vi "AnalogIntegrator_NI5751.vi"() -> ()   [LabVIEW 2012]
uses:
  <vilib>/Platform/TimedLoop/XDataNode/timing_clust.ctl
  <vilib>/Platform/TimedLoop/XDataNode/nitl_modes.ctl
  <vilib>/Platform/TimedLoop/XDataNode/wakeup.ctl
  <vilib>/rvi/eio/common/nirviEmuTemplateMethod_errors.vi
  <vilib>/rvi/FIFO/Fifo_Resource/nirvififoEmulationSetSize.vi
  <vilib>/rvi/DataTransferAndStorage/Container/Common/niFpgaContainerGetUniqueNameForEmu.vi
  <vilib>/rvi/Emulation/niFpgaSctlEmulationRegisterWithScheduler.vi
  <vilib>/rvi/errors/niFpgaSetErrorForExecOnDevCompSimple.vi
  <vilib>/rvi/eio/common/nirviEmuReportErrorAndStop.vi
  <vilib>/rvi/Emulation/niFpgaSctlEmulationFifoFullMgr.vi
  <vilib>/rvi/Emulation/niFpgaSctlEmulationResourceMgr.vi
  <vilib>/rvi/Emulation/niFpgaSctlEmulationScheduler.vi
  <vilib>/rvi/interface/RandomDataEmulation/nirviRandomDataFPGAFIFO.vi
  <vilib>/rvi/interface/RandomDataEmulation/niFpgaRandomDataHandleErrors.vi
  <vilib>/rvi/Emulation/niFpgaSctlEmulationGlobalWrite.vi
  <vilib>/Platform/TimedLoop/XDataNode/XDataNode.xnode
  <vilib>/eio/EIONode/EIONode.xnode
  <vilib>/rvi/DataTransferAndStorage/Container/XNode/niFpgaContainer.xnode
  <vilib>/rvi/FIFO/Fifo_Resource/nirvififoEmulationClear.vi
  <vilib>/rvi/FIFO/Fifo_Resource/nirvififoEmulationWrite.vi
  <vilib>/rvi/FIFO/Fifo_Resource/nirvififoEmulationRead.vi
  <vilib>/rvi/interface/RandomDataEmulation/nirviRandomDataFpgaReadWriteTemplate.vi
  <vilib>/Platform/TimedLoop/XDataNode/XDNodeRunTimeDep.lvlib
panel:
  in  "Baselinex8 Ch2":u16
  in  "Baselinex8 Ch1":u16
  in  "Clear Interloop FIFO":bool
  out "InterloopFIFO Timeout":bool
  out "ToHostCh2FIFO Overflow":bool
  out "ToHostCh1FIFO Overflow":bool
  out "Pixel counter":u32
  in  "Wait for trigger":bool
  in  "Acquire":bool
  in  "Acquire continuously":bool=TRUE
  in  "Requested pixels":u32=100000
  out "InterloopFIFO Overflow":bool
  out "Acquiring":bool
  out "IO Module\\AI Over Range":bool
  in  "Samples per pixel":u32=10000 caption="Samples per pixel Acq"
  in  "Samples per line":u32=10000 caption="Samples per pixel Acq"
  out "Configured?":bool
  # "5771 IO module configuration"
  # "Analog integrator"
  # "Acquisition control"
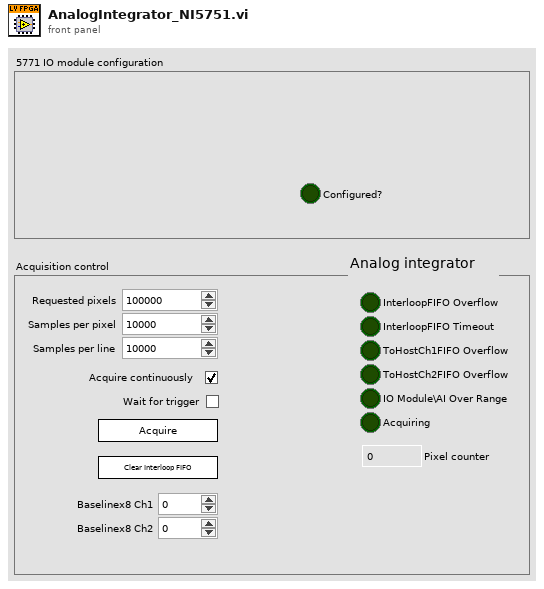
[diagram p1: front panel]
types:
  T1 = typedef "XDNodeRunTimeDep.lvlib/timing_clust.ctl" = cluster{"Expected End [f-1]":u64, "Actual End [f-1]":u64, "Finished Late? [f-1]":bool, "Expected End [i-1]":u64, "Actual End [i-1]":u64, "Finished Late? [i-1]":bool, "Expected Start [i]":u64, "Actual Start [i]":u64, "Expected Start [f]":u64, "Actual Start [f]":u64, "Source Name":string, "Structure Name":string, "Period":i64, "Deadline":i64, "Offset":i64, "Start":i64, "Priority":i32, "Timeout":i32, "Mode":T2, "Wakeup Reason":T3, "Error":errorcluster, "Source Type":string, "Secondary Source Type":string, "Global End Time":u64, "Global Start Time":u64, "Frame Duration":u64, "Iteration Duration":u64, "Assigned CPU":i32, "I/O Scan Engine Mode":u32}
  T2 = typedef "XDNodeRunTimeDep.lvlib/nitl_modes.ctl" = enum32{"No Change", "Process missed periods, maintain original phase", "Discard missed periods, maintain original phase", "Process missed periods, ignore original phase", "Discard missed periods, ignore original phase"}
  T3 = typedef "XDNodeRunTimeDep.lvlib/wakeup.ctl" = enum32{"Normal", "Aborted", "Asynchronous wakeup", "Timing source error", "Timed loop error", "Timeout"}
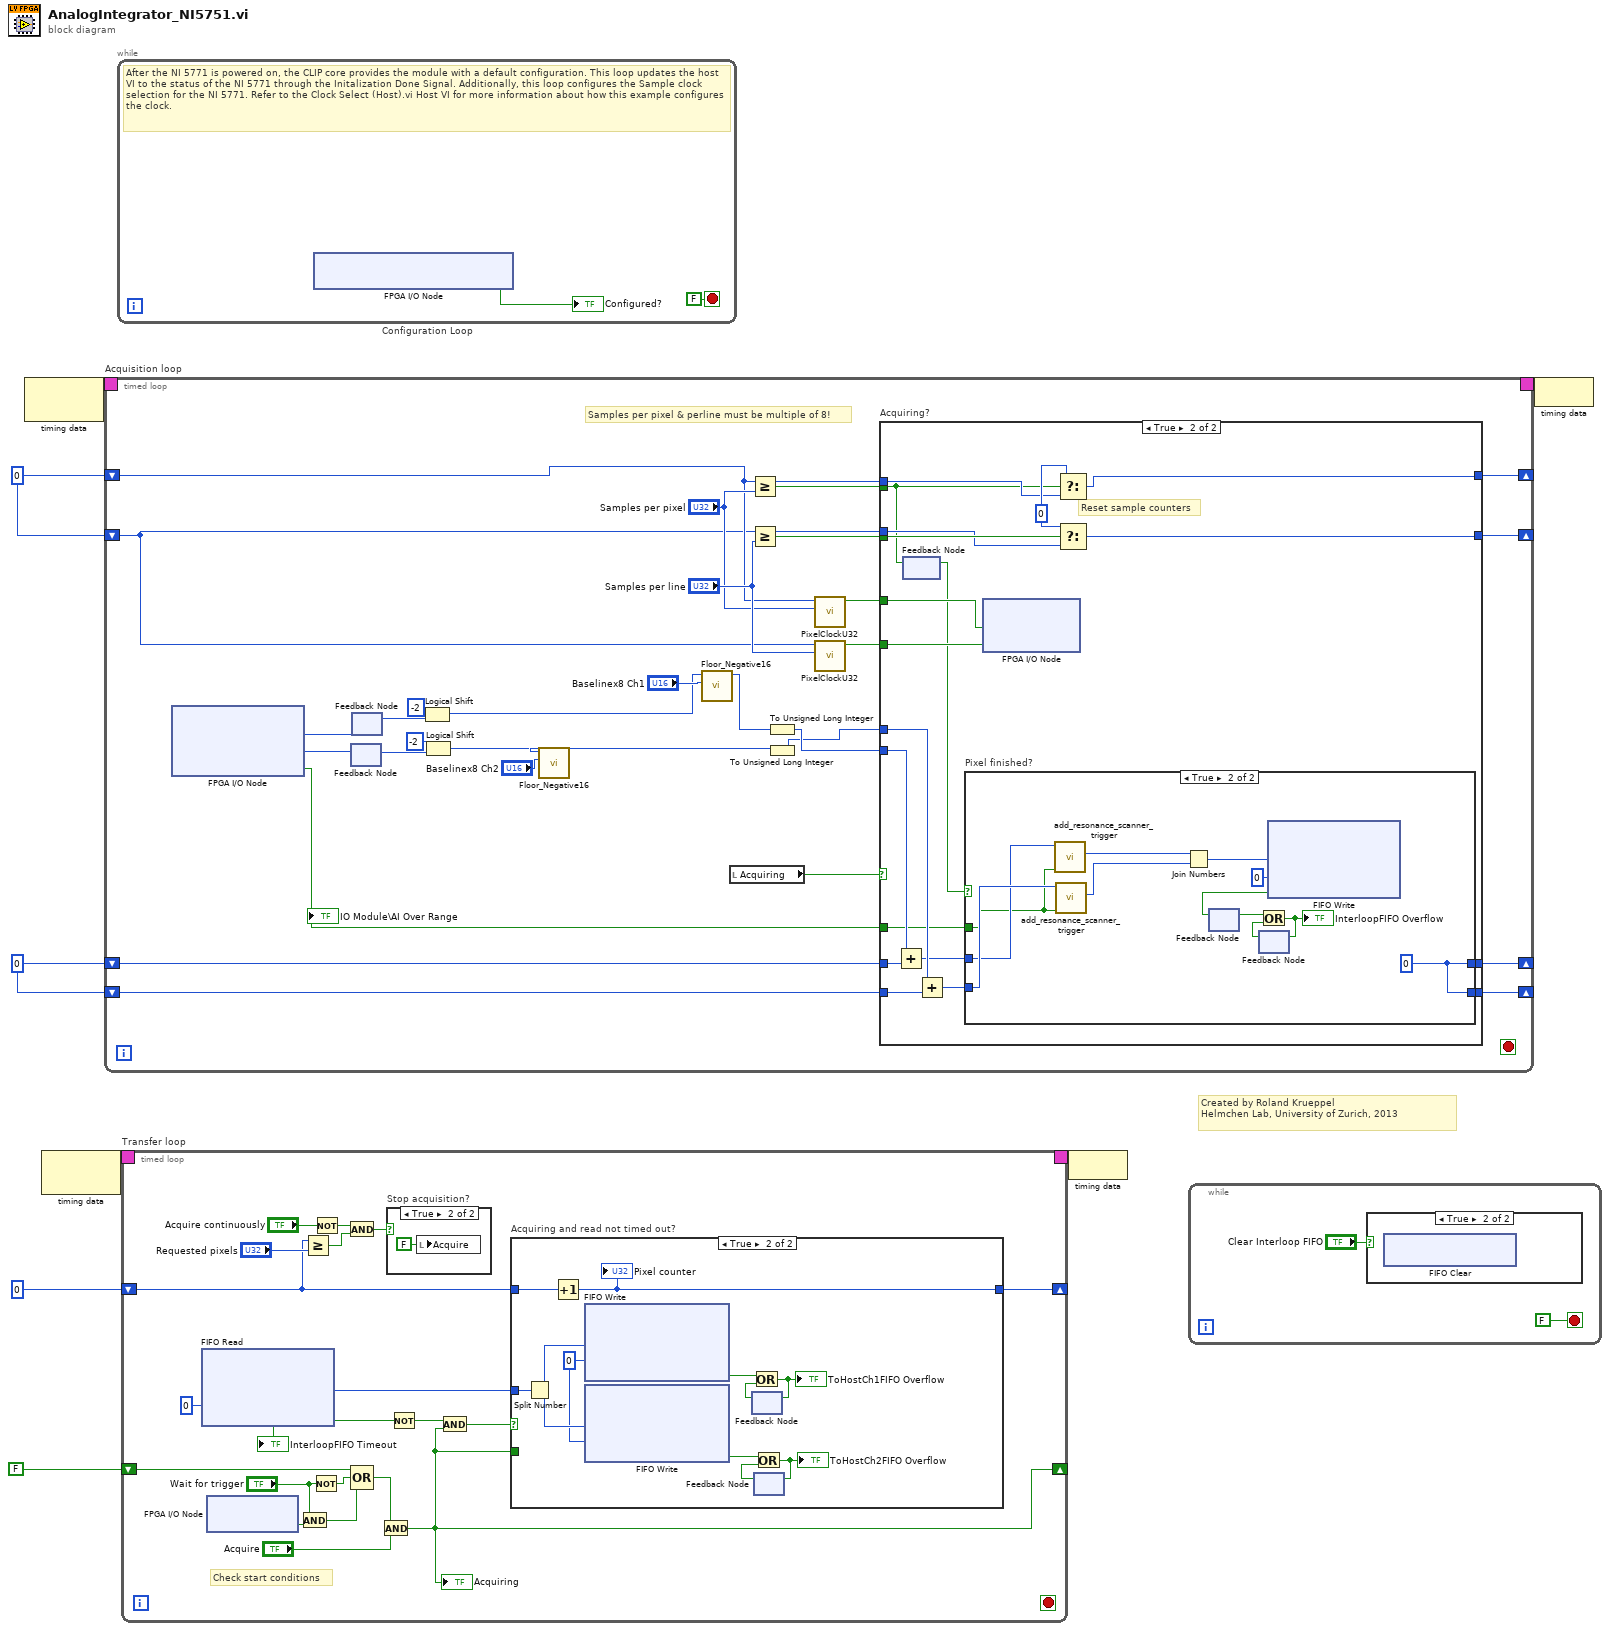
[diagram p0: block diagram]
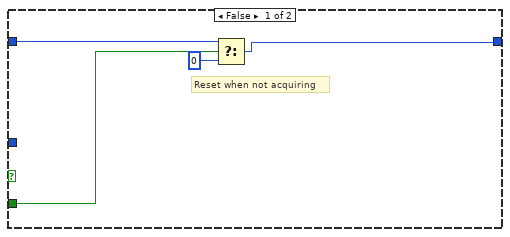
[diagram p4: hidden frame]
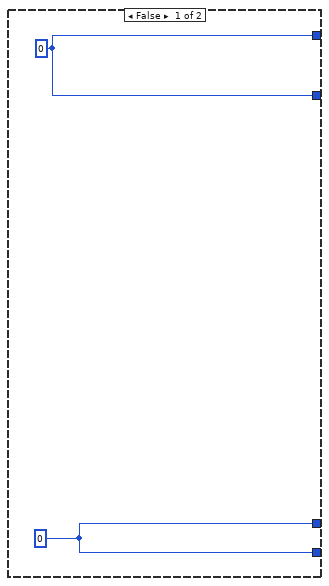
[diagram p5: hidden frame]
diagram:
  w5 = u32 0
  w6 = u32 0 ("t")
  # "Created by Roland Krueppel\nHelmchen Lab, University of Zurich, 2013"
  n1 = node-c288() -> (w8:T1)  [unwired: 1 in]
  n2 = node-c288() -> (w4:T1)  [unwired: 1 in]
  n3 = timed-loop "Acquisition loop" {
    timing: w8 -> [_]
    timing-out: [_] -> w7
    shift-right: [w37] -> _
    shift-left: w6 -> [w21]
    shift-right: [w38] -> _
    shift-left: w6 -> [w22]
    shift-right: [w33] -> _
    shift-left: w5 -> [w35]
    shift-right: [w32] -> _
    shift-left: w5 -> [w34]
    stop <- _ stop-if-true
    # "Samples per pixel & perline must be multiple of 8!"
    n4 = xnode "FPGA I/O Node"() -> ("IO Module\\AI A0"=w25:i16, "IO Module\\AI A1"=w24:i16, "IO Module\\DI 0"=w23:bool)  [unwired: 3 in, 3 out]
    n5 = feedback #1() -> (w16:i16)  [unwired: 1 in]
    n6 = feedback-in #1(w24) -> ()
    n7 = feedback-in #2(w25) -> ()
    n8 = feedback #2() -> (w11:i16)  [unwired: 1 in]
    n9 = Logical Shift(y=i16 -2, x=w11) -> (x << y=w12:i16)
    n10 = Logical Shift(y=i16 -2, x=w16) -> (x << y=w14:i16)
    n11 = call "Floor_Negative16.vi"("Baseline U16"="Baselinex8 Ch2", "Input Value"=w14) -> ("Output Value"=w19:u16)  [unwired: 9 in]
    n12 = call "Floor_Negative16.vi"("Baseline U16"="Baselinex8 Ch1", "Input Value"=w12) -> ("Output Value"=w20:u16)  [unwired: 9 in]
    n13 = local read "Acquiring"() -> (w36:bool)
    n14 = Greater Or Equal?(x=w22, y="Samples per pixel") -> (x >= y?=w27:bool)
    n15 = Greater Or Equal?(x=w21, y="Samples per line") -> (x >= y?=w26:bool)
    n16 = To Unsigned Long Integer(number=w20) -> (unsigned 32bit integer=w10:u32)
    n17 = To Unsigned Long Integer(number=w19) -> (unsigned 32bit integer=w9:u32)
    n18 = call "PixelClockU32.vi"("Samples per pixel"="Samples per pixel", "Sample counter"=w22) -> ("Pixel clock"=w29:bool)  [unwired: 9 in]
    n19 = call "PixelClockU32.vi"("Samples per pixel"="Samples per line", "Sample counter"=w21) -> ("Pixel clock"=w28:bool)  [unwired: 9 in]
    n20 = case "Acquiring?" shown="True" w36 {
      tunnel: [w40 w58] -> w38
      tunnel: [w40 w57] -> w37
      tunnel: w10 -> [_ w55]
      tunnel: w35 -> [_ w56]
      tunnel: w34 -> [_ w54]
      tunnel: w9 -> [_ w53]
      tunnel: [w39 w50] -> w33
      tunnel: [w39 w49] -> w32
      tunnel: w27 -> [_ w43]
      tunnel: w26 -> [_ w48]
      tunnel: w22 -> [_ w47]
      tunnel: w21 -> [_ w46]
      tunnel: w29 -> [_ w45]
      tunnel: w28 -> [_ w44]
      tunnel: w23 -> [_ w41]
      frame False {
        w39 = u32 0
        w40 = u16 0 ("t")
      }
      frame True {
        w59 = u32 0 ("t")
        # "Reset sample counters"
        n21 = Add(x=w55, y=w56) -> (x+y=w51:u32)
        n22 = feedback #3() -> (w42:bool)  [unwired: 1 in]
        n23 = feedback-in #3(w43) -> ()
        n24 = Add(x=w53, y=w54) -> (x+y=w52:u32)
        n25 = case "Pixel finished?" shown="True" w42 {
          tunnel: w52 -> [w60 w66]
          tunnel: w51 -> [w61 w65]
          tunnel: [w61 w69] -> w50
          tunnel: [w60 w69] -> w49
          tunnel: w41 -> [_ w64]
          frame False {
          }
          frame True {
            w69 = u32 0
            n26 = call "add_resonance_scanner_trigger.vi"("Trigger"=w64, "Input"=w65) -> ("Output"=w63:u32)  [unwired: 9 in]
            n27 = call "add_resonance_scanner_trigger.vi"("Trigger"=w64, "Input"=w66) -> ("Output"=w62:u32)  [unwired: 9 in]
            n28 = Join Numbers(hi=w63, lo=w62) -> ((hi.lo)=w73:u64)
            n29 = feedback #4() -> (w68:bool)  [unwired: 1 in]
            n30 = feedback #5() -> (w70:bool)  [unwired: 1 in]
            n31 = Or(x=w68, y=w70) -> (x .or. y?=w71:bool)
            "InterloopFIFO Overflow" <- w71
            n32 = feedback-in #5(w71) -> ()
            n33 = xnode ("FIFO Write")("Element"=w73, "Timeout"=0) -> ("Timed Out?"=w67:bool)  [unwired: 1 in, 1 out]
            n34 = feedback-in #4(w67) -> ()
          }
        }
        n35 = xnode "FPGA I/O Node"("PixelClock"=w45, "LineClock"=w44) -> ()  [unwired: 2 in, 2 out]
        n36 = Select(t=w59, s=w43, f=w47) -> (s? t:f=w58:u32)
        n37 = Select(t=w59, s=w48, f=w46) -> (s? t:f=w57:u32)
      }
    }
  }
  n38 = while "Configuration Loop" {
    stop <- FALSE stop-if-true
    # "After the NI 5771 is powered on, the CLIP core provides the module with a default configuration. This loop updates the host VI to the status of the NI 5771 through the Initalization Done Signal. Additionally, this loop configures the Sample clock selection for the NI 5771. Refer to the Clock Select (Host).vi Host VI for more information about how this example configures the clock."
    n39 = xnode "FPGA I/O Node"() -> ("IO Module\\Initialization Done"=→"Configured?":bool)  [unwired: 1 in, 1 out]
  }
  n40 = timed-loop "Transfer loop" {
    timing: w4 -> [_]
    timing-out: [_] -> w3
    shift-right: [w80] -> _
    shift-left: u32 0 -> [w81]
    shift-right: [w79] -> _
    shift-left: FALSE -> [w87]
    stop <- _ stop-if-true
    # "Check start conditions"
    n41 = xnode ("FIFO Read")("Timeout"=0) -> ("Element"=w82:u64, "Timed Out?"=w86:bool)  [unwired: 1 in, 1 out]
    "InterloopFIFO Timeout" <- w86
    n42 = xnode "FPGA I/O Node"() -> ("TriggerIn"=w92:bool)  [unwired: 1 in, 1 out]
    n43 = And(x="Wait for trigger", y=w92) -> (x .and. y?=w89:bool)
    n44 = Greater Or Equal?(x=w81, y="Requested pixels") -> (x >= y?=w94:bool)
    n45 = Not(x="Wait for trigger") -> (.not. x?=w90:bool)
    n46 = Not(x="Acquire continuously") -> (.not. x?=w95:bool)
    n47 = And(x=w95, y=w94) -> (x .and. y?=w84:bool)
    n48 = Compound Arithmetic op=OR(w87, w90, w89) -> (w88:bool)
    n49 = And(x=w88, y="Acquire") -> (x .and. y?=w79:bool)
    "Acquiring" <- w79
    n50 = case "Stop acquisition?" shown="True" w84 {
      frame False {
      }
      frame True {
        n51 = local write "Acquire"(FALSE ("Acquire")) -> ()
      }
    }
    n52 = Not(x=w86) -> (.not. x?=w85:bool)
    n53 = And(x=w85, y=w79) -> (x .and. y?=w83:bool)
    n54 = case "Acquiring and read not timed out?" shown="True" w83 {
      tunnel: w82 -> [_ w114]
      tunnel: w81 -> [w101 w110]
      tunnel: [w100 w109] -> w80
      tunnel: w79 -> [w102 _]
      frame False {
        # "Reset when not acquiring"
        n55 = Select(t=w101, s=w102, f=u32 0) -> (s? t:f=w100:u32)
      }
      frame True {
        w111 = 0 ("Timeout")
        n56 = Split Number(x=w114) -> (hi(x)=w113:u32, lo(x)=w112:u32)
        n57 = Increment(x=w110) -> (x+1=w109:u32)
        "Pixel counter" <- w109
        n58 = xnode ("FIFO Write")("Element"=w113, "Timeout"=w111) -> ("Timed Out?"=w107:bool)  [unwired: 1 in, 1 out]
        n59 = xnode ("FIFO Write")("Element"=w112, "Timeout"=w111) -> ("Timed Out?"=w104:bool)  [unwired: 1 in, 1 out]
        n60 = feedback #6() -> (w106:bool)  [unwired: 1 in]
        n61 = Or(x=w107, y=w106) -> (x .or. y?=w108:bool)
        "ToHostCh1FIFO Overflow" <- w108
        n62 = feedback-in #6(w108) -> ()
        n63 = feedback #7() -> (w103:bool)  [unwired: 1 in]
        n64 = Or(x=w104, y=w103) -> (x .or. y?=w105:bool)
        "ToHostCh2FIFO Overflow" <- w105
        n65 = feedback-in #7(w105) -> ()
      }
    }
  }
  n66 = node-c288(w3) -> ()
  n67 = while {
    stop <- FALSE stop-if-true
    n68 = case shown="True" "Clear Interloop FIFO" {
      frame False {
      }
      frame True {
        n69 = xnode ("FIFO Clear")() -> ()  [unwired: 1 in, 1 out]
      }
    }
  }
  n70 = node-c288(w7) -> ()
